vi "ErrorManager.vi"(3 "error in (no error)":errorcluster {"code" format="%x"}, 5 "error code":i32 format="%x") -> (0 "error out":errorcluster {"code" format="%x"})   [LabVIEW 2019]
doc: "ErrorManager tranlsates error numbers generated by the pco.camera interface into language. Information on the source of the error, the device and software layer where the error originated is coded into the error string. \nThis function is called by all SDK and recorder SDK functions, so that error numbers can be converted into LabVIEW error clusters for further handling."
panel:
  out "statusError":bool
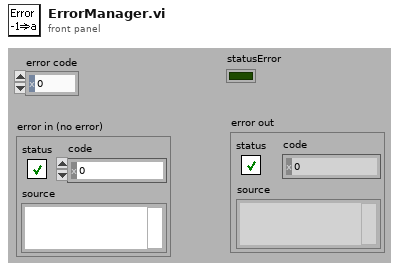
[diagram p1: front panel]
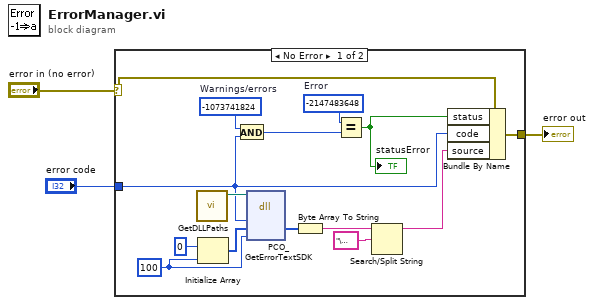
[diagram p0: block diagram]
diagram:
  n1 = case shown="No Error" "error in (no error)" {
    selector: "error in (no error)" -> [w9 w19]
    tunnel: [w11 w19] -> w1
    tunnel: "error code" -> [w6 _]
    frame No Error {
      w7 = -2147483648  # Error
      w8 = -1073741824  # Warnings/errors
      w16 = u32 100 ("dimension size")
      n2 = call "GetDLLPaths.vi"() -> ("SC2_Cam_Path"=w10:path)  [unwired: 9 in, 2 out]
      n3 = Initialize Array(u8 0, w16) -> (w17:u8[])
      n4 = And(x=w8, y=w6) -> (x .and. y?=w5:i32)
      n5 = dll-call lib="?" fn="PCO_GetErrorTextSDK"(path in=w10, "errorCode"=w6, "pBuf"=w17, "bufLength"=w16) -> ("pBuf"=w14:u8[])  [unwired: 5 in, 2 out]
      n6 = Byte Array To String(unsigned byte array=w14) -> (string=w15:string)
      n7 = Equal?(x=w7, y=w5) -> (x = y?=w4:bool)
      "statusError" <- w4
      n8 = Search/Split String(string=w15, search string/char (-)="\u0000" ("search string")) -> (substring before match=w12:string)  [unwired: 1 in, 2 out]
      n9 = Bundle By Name(cluster=w9, "status"=w4, "code"=w6, "source"=w12) -> (w11:errorcluster)
    }
    frame Error {
    }
  }
  "error out" <- w1
